vi "Get File Infor.vi"(8 "error in (no error)":errorcluster, 11 "TDMS in":refnum<class "TDMS.lvclass">) -> (0 "error out":errorcluster, 3 "TDMS out":refnum<class "TDMS.lvclass">)   [LabVIEW 2020, in "TDMS.lvclass"]
uses:
  TDMS.lvclass
  TDMS.lvclass/TDMS.ctl
  Abstrut Data/Abstruct Data Type.lvclass/Abstruct Data Type.ctl
  cc793d6c-822d-460a-9e93-0fe597a351d8.vi
  Abstrut Data/Accessors/Write All Channels.vi
  Abstrut Data/Accessors/Write Length.vi
  Abstrut Data/Accessors/Write Table Names.vi
  cc793d6c-822d-460a-9e93-0fe597a351d8.vi/d4db2432-cc9c-482c-8957-dac855435ef6.vi
  cc793d6c-822d-460a-9e93-0fe597a351d8.vi/86fbf154-bd7b-49a2-8ab2-a837b2a95f24.vi
  cc793d6c-822d-460a-9e93-0fe597a351d8.vi/3b95b01e-1ec2-4565-bcd9-7606a5281010.vi
  cc793d6c-822d-460a-9e93-0fe597a351d8.vi/96a08935-737a-44b2-979c-a81d56408f7e.vi
  cc793d6c-822d-460a-9e93-0fe597a351d8.vi/d4db2432-cc9c-482c-8957-dac855435ef6.vi/6eaecd13-6e48-4772-a921-b51ebdf84d88.vi
  cc793d6c-822d-460a-9e93-0fe597a351d8.vi/d4db2432-cc9c-482c-8957-dac855435ef6.vi/d2d5f2b7-06f4-47f6-971c-049c3fdbb653.vi
  cc793d6c-822d-460a-9e93-0fe597a351d8.vi/3b95b01e-1ec2-4565-bcd9-7606a5281010.vi/6eaecd13-6e48-4772-a921-b51ebdf84d88.vi
  cc793d6c-822d-460a-9e93-0fe597a351d8.vi/3b95b01e-1ec2-4565-bcd9-7606a5281010.vi/d2d5f2b7-06f4-47f6-971c-049c3fdbb653.vi
  cc793d6c-822d-460a-9e93-0fe597a351d8.vi/96a08935-737a-44b2-979c-a81d56408f7e.vi/6eaecd13-6e48-4772-a921-b51ebdf84d88.vi
  cc793d6c-822d-460a-9e93-0fe597a351d8.vi/96a08935-737a-44b2-979c-a81d56408f7e.vi/d2d5f2b7-06f4-47f6-971c-049c3fdbb653.vi
  <vilib>/Comparison/Less/Less Functor/Less Functor.lvclass
  Abstrut Data/Abstruct Data Type.lvclass
panel:
  out "Cnannel Names":string[](array[string])
  out "file contents":cluster{string, string[]}[](array[cluster])
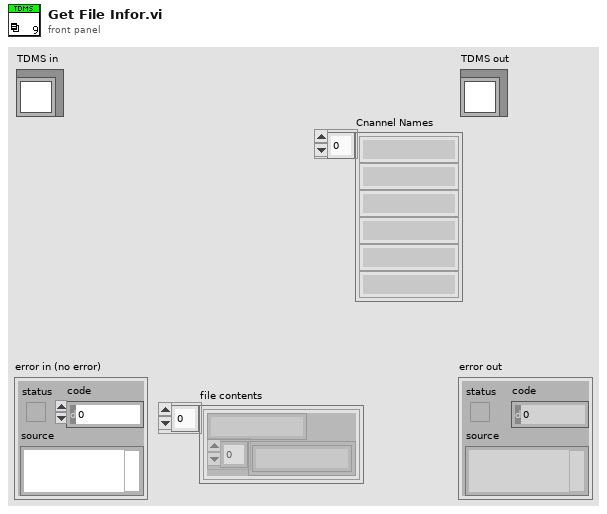
[diagram p1: front panel]
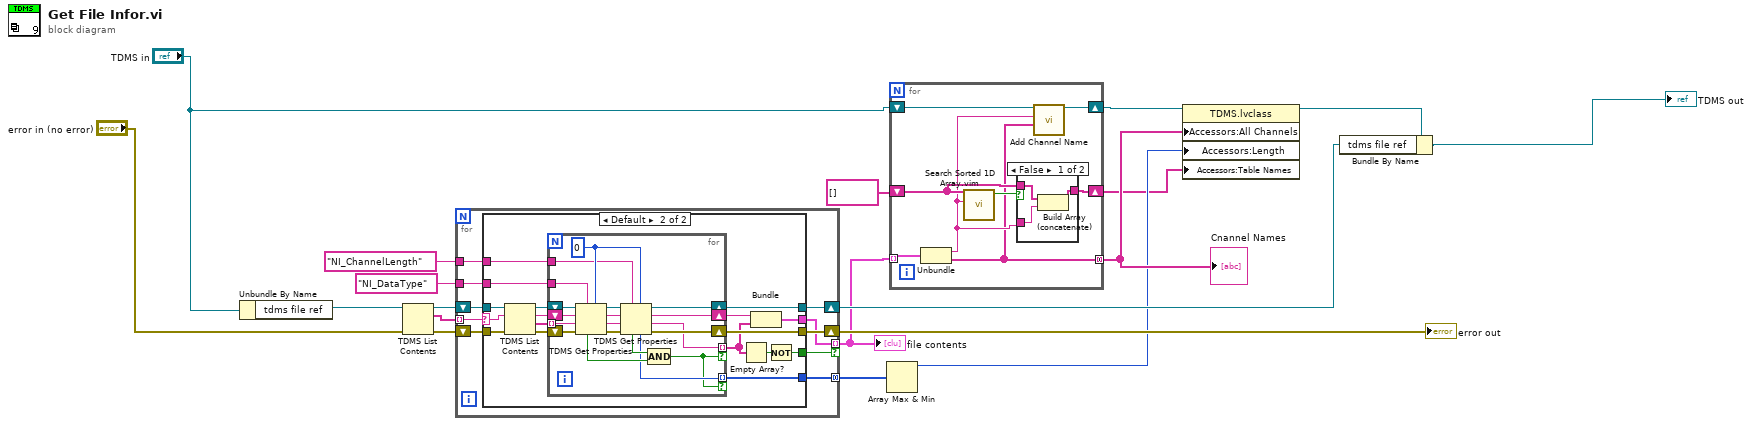
[diagram p0: block diagram]
diagram:
  n1 = Unbundle By Name("TDMS in") -> ("tdms file ref"=w14:refnum<k34>)
  n2 = TDMS List Contents(4:"error in (no error)", 7:w14) -> (0:w19:errorcluster, 2:w16:string[], 3:w15:refnum<k34>)  [unwired: 1 in, 1 out]
  n3 = for {
    tunnel: w16 -> [w27] mode=indexing
    shift-right: [w25] -> w11
    shift-left: w15 -> [w26]
    shift-right: [w28] -> w12
    shift-left: w19 -> [w29]
    tunnel: [w23] -> w10 mode=indexing if=w24
    tunnel: "NI_ChannelLength" ("property name") -> [w22]
    tunnel: "NI_DataType" ("property name") -> [w21]
    tunnel: [w20] -> w8 mode=concatenating
    n4 = case shown="Default" w27 {
      selector: w27 -> [_ w45]
      tunnel: w26 -> [w30 w44]
      tunnel: [w30 w39] -> w25
      tunnel: w29 -> [w31 w48]
      tunnel: [w31 w46] -> w28
      tunnel: [_ w42] -> w24
      tunnel: [_ w41] -> w23
      tunnel: w22 -> [_ w36]
      tunnel: w21 -> [_ w35]
      tunnel: [_ w32] -> w20
      frame "" {
      }
      frame Default {
        n5 = TDMS List Contents(4:w48, 6:w45, 7:w44) -> (0:w47:errorcluster, 1:w37:string[], 2:w38:string, 3:w40:refnum<k34>)
        n6 = for {
          shift-right: [w53] -> w39
          shift-left: w40 -> [w64]
          shift-right: [w65] -> w46
          shift-left: w47 -> [w67]
          tunnel: w37 -> [w62] mode=indexing
          shift-right: [w58] -> w33
          shift-left: w38 -> [w63]
          tunnel: [w57] -> w34 mode=indexing if=w49
          tunnel: w36 -> [w55]
          tunnel: w35 -> [w54]
          tunnel: [w50] -> w32 mode=indexing if=w49
          w56 = u16 0
          n7 = TDMS Get Properties(5:w56, 7:w54, 8:w67, 9:w62, 10:w63, 11:w64) -> (0:w66:errorcluster, 1:w60:string, 2:w61:string, 3:w59:refnum<k34>, 6:w51:bool)  [unwired: 1 out]
          n8 = TDMS Get Properties(5:w56, 7:w55, 8:w66, 9:w60, 10:w61, 11:w59) -> (0:w65:errorcluster, 1:w57:string, 2:w58:string, 3:w53:refnum<k34>, 4:w50:u16, 6:w52:bool)
          n9 = Compound Arithmetic op=AND(w52, w51) -> (w49:bool)
        }
        n10 = Empty Array?(array=w34) -> (empty?=w43:bool)
        n11 = Bundle(w33, w34) -> (w41:cluster{string, string[]})  [unwired: 1 in]
        n12 = Not(x=w43) -> (.not. x?=w42:bool)
      }
    }
  }
  "error out" <- w12
  "file contents" <- w10
  n13 = Array Max & Min(array=w8) -> (max value=w7:u16)  [unwired: 3 out]
  n14 = for {
    tunnel: w10 -> [w75] mode=indexing
    tunnel: [w68] -> w9 mode=concatenating
    shift-right: [w72] -> w5
    shift-left: string[] [] ("Table Names") -> [w73]
    shift-right: [w71] -> w4
    shift-left: "TDMS in" -> [w70]
    n15 = Unbundle(w75) -> (w69:string, w68:string[])
    n16 = call "Search Sorted 1D Array.vim"("element"=w69, "sorted 1D array"=w73) -> ("found?"=w74:bool)  [unwired: 8 in, 1 out]
    n17 = case shown="False" w74 {
      tunnel: w69 -> [w77 _]
      tunnel: w73 -> [w78 w79]
      tunnel: [w76 w79] -> w72
      frame False {
        n18 = Build Array (concatenate)(w78, w77) -> (w76:string[])
      }
      frame True {
      }
    }
    n19 = call "Add Channel Name.vi"("Channel Names"=w68, "Table Name"=w69, "Abstruct Data Type in"=w70) -> ("Abstruct Data Type out"=w71:refnum<class "TDMS.lvclass">)  [unwired: 7 in, 1 out]
  }
  "Cnannel Names" <- w9
  n20 = property class="TDMS.lvclass"(reference=w4, "Accessors:All Channels"=w9, "Accessors:Length"=w7, "Accessors:Table Names"=w5) -> (reference out=w2:refnum<class "TDMS.lvclass">)  [unwired: 1 in, 1 out]
  n21 = Bundle By Name(cluster=w2, "tdms file ref"=w11) -> (→"TDMS out":refnum<class "TDMS.lvclass">)
